vi "CLD 13 Flow Rates Exercise.vi"() -> ()   [LabVIEW 2025]
doc: "CLD 13 exercise"
uses:
  CLD 13 State Machine Enum.ctl
  CLD 13 Data Cluster.ctl
  CLD 13 timer Enum.ctl
panel:
  out "Elapsed Time":dbl
  out "Flow Rate Meter":i8(knob) scale=-20.0..20.0 scale format="%_2f"
  out "Flow Rate":dbl
  out "Error Out":errorcluster
  in  "Error In":errorcluster
  in  "Stop Application":bool
  in  "Stop Flow":bool
  in  "Flow Rate Change":i8(slide) min=-2 max=2 step=1 scale=-2.0..2.0
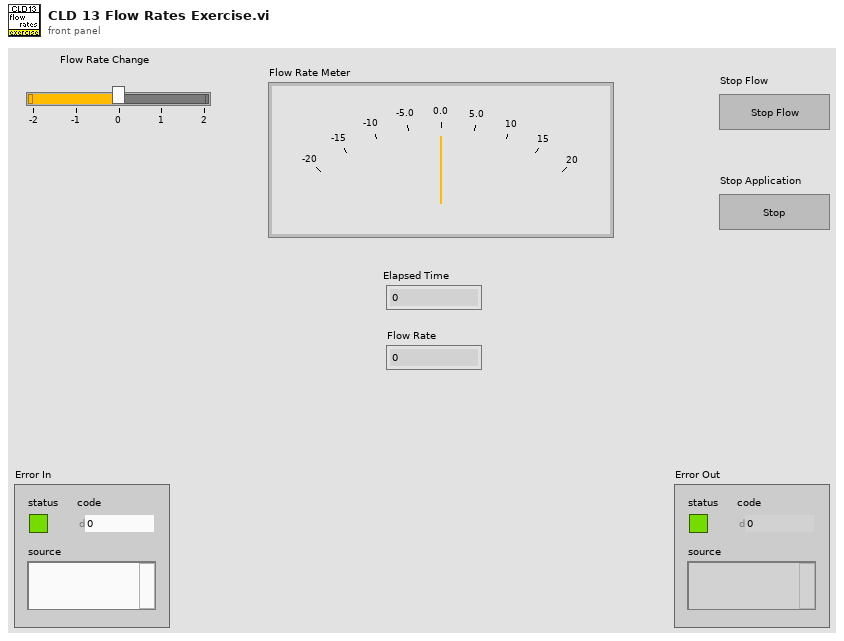
[diagram p1: front panel]
types:
  T1 = typedef "CLD 13 Data Cluster.ctl" = cluster{"Flow Rate Change":i8, "Flow Rate":i8}
  T2 = typedef "CLD 13 State Machine Enum.ctl" = enum16{"Initialize", "Idle", "Stop Flow", "Process"}
  T3 = cluster{"Cluster":T1, "Flow Rate Target":i8, "Operation Mode":enum16{"Normal", "Stop Flow"}}
  T4 = typedef "CLD 13 timer Enum.ctl" = enum16{"Start", "Read"}
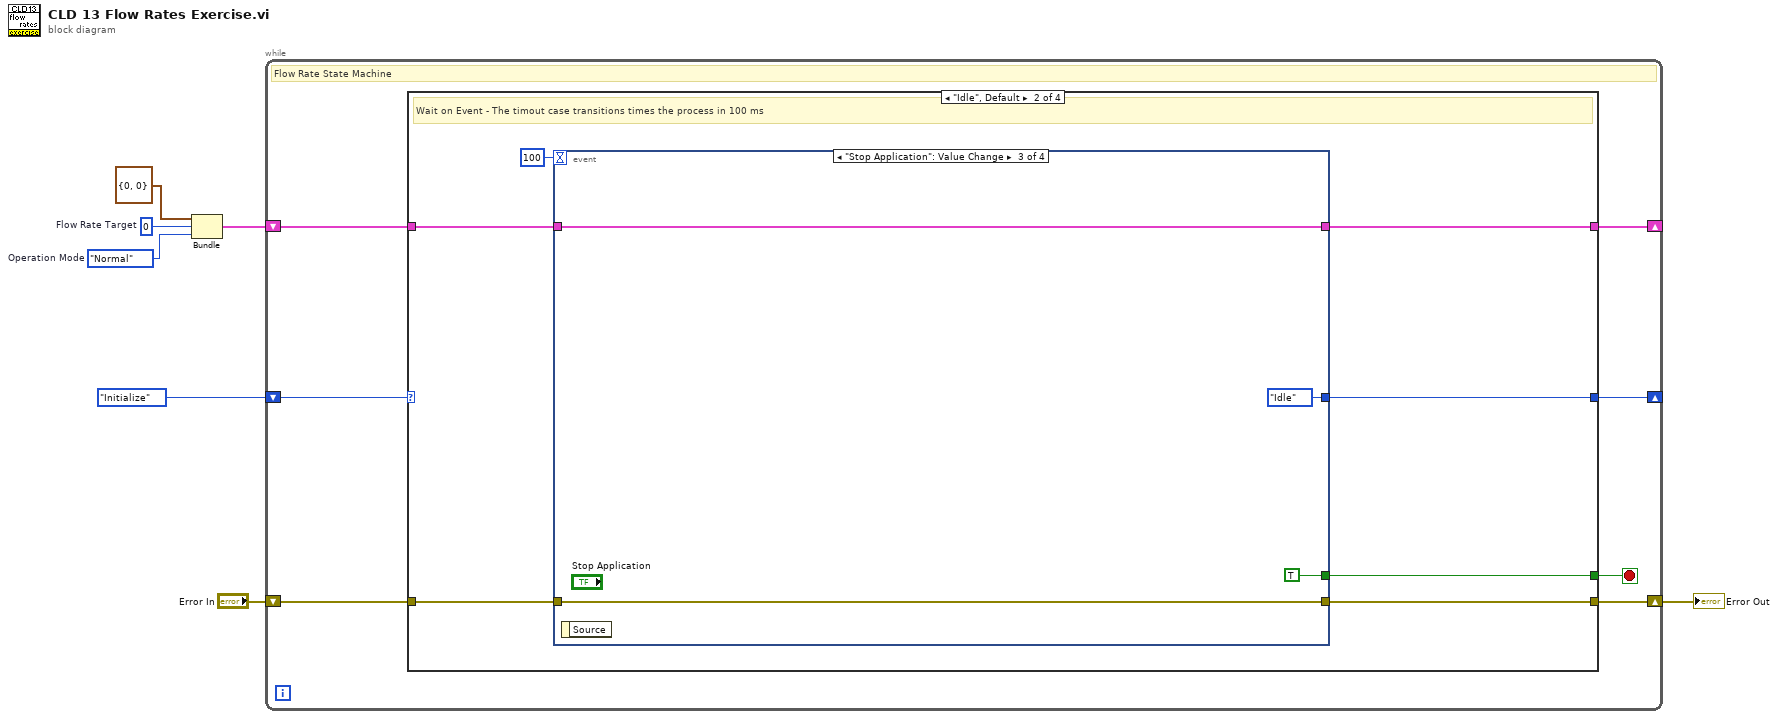
[diagram p0: block diagram]
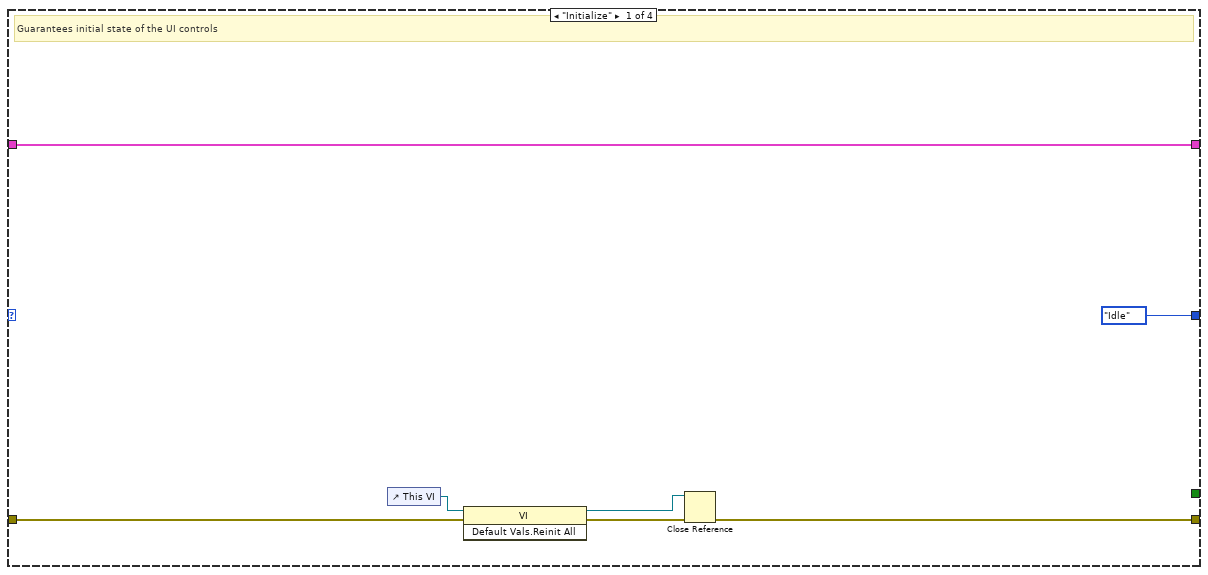
[diagram p2: hidden frame]
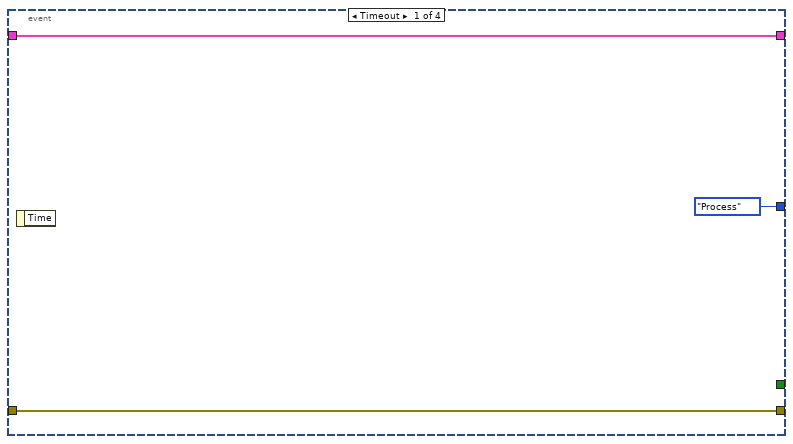
[diagram p3: hidden frame]
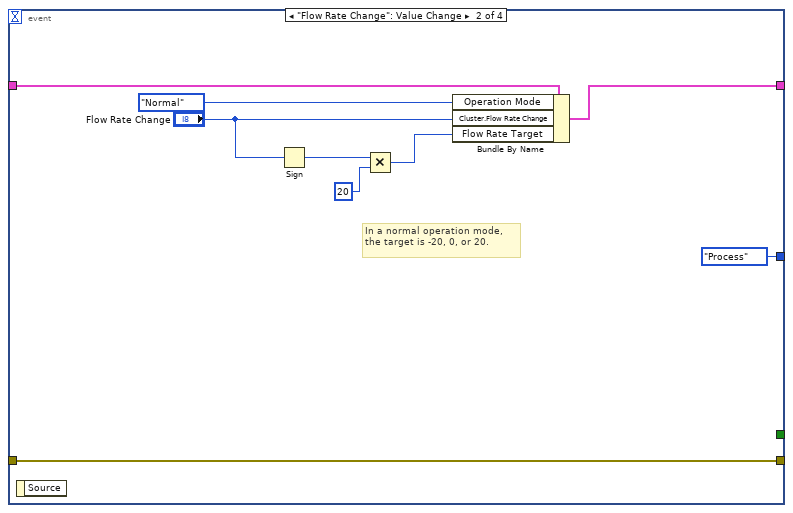
[diagram p4: hidden frame]
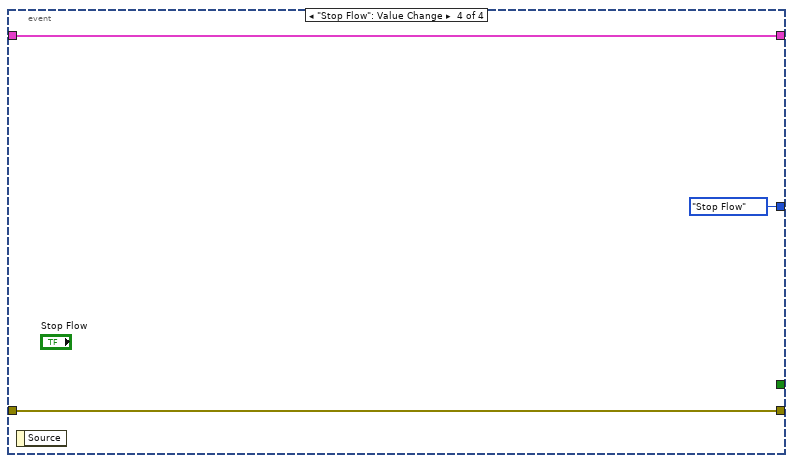
[diagram p5: hidden frame]
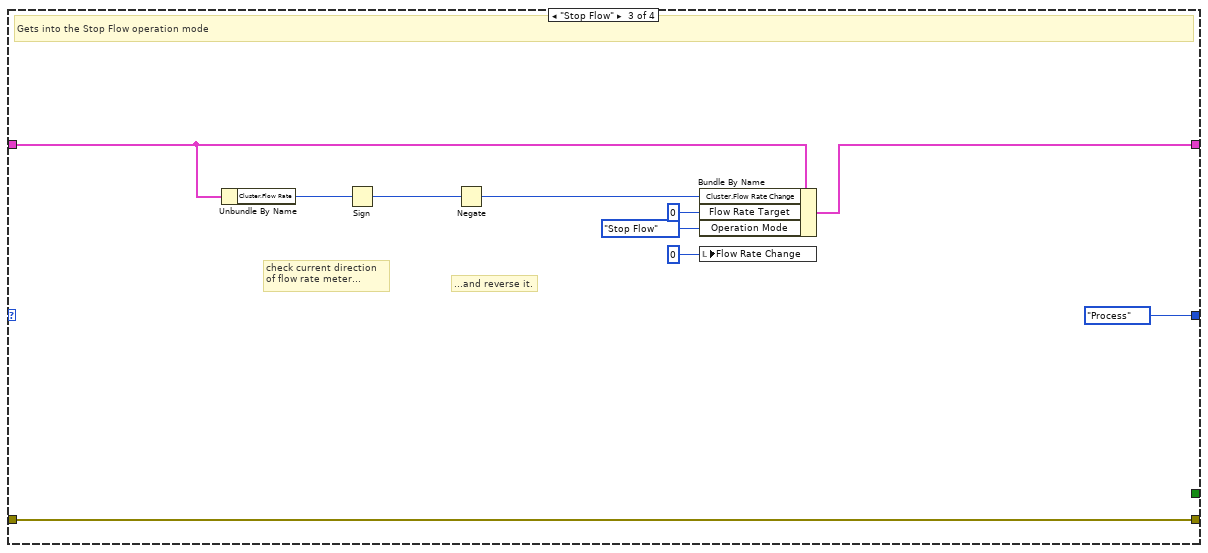
[diagram p6: hidden frame]
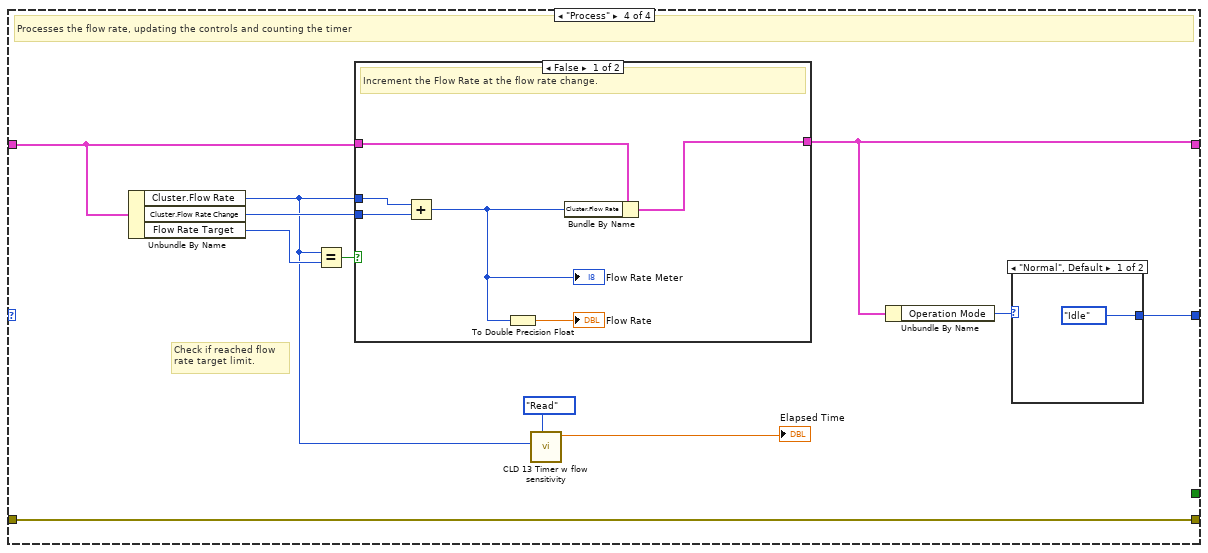
[diagram p7: hidden frame]
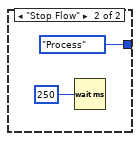
[diagram p8: hidden frame]
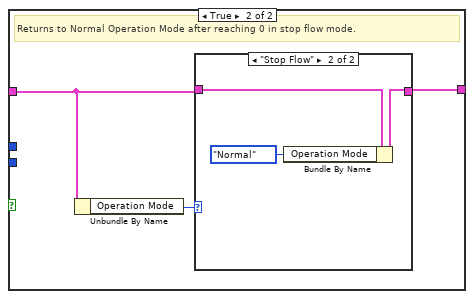
[diagram p9: hidden frame]
diagram:
  w1 = enum16{"Normal", "Stop Flow"}."Normal"  # Operation Mode
  w3 = i8 0  # Flow Rate Target
  n1 = Bundle("Cluster"=T1 {"Flow Rate Change"=0, "Flow Rate"=0}, "Flow Rate Target"=w3, "Operation Mode"=w1) -> (w2:T3)  [unwired: 1 in]
  n2 = while {
    shift-right: [w13] -> w6
    shift-left: "Error In" -> [w14]
    shift-right: [w10] -> _
    shift-left: w2 -> [w11]
    shift-right: [w9] -> _
    shift-left: CLD_13_State_Machine_Enum."Initialize" ("CLD 13") -> [w12]
    stop <- w8 stop-if-true
    # "Flow Rate State Machine"
    n3 = case shown="\"Idle\", Default" w12 {
      tunnel: w14 -> [w21 w28 w57 w68]
      tunnel: [w18 w25 w57 w68] -> w13
      tunnel: w11 -> [w20 w23 w52 w61]
      tunnel: [w20 w26 w51 w62] -> w10
      tunnel: [CLD_13_State_Machine_Enum."Idle" ("CLD 13") w27 CLD_13_State_Machine_Enum."Process" ("CLD 13") w59] -> w9
      tunnel: [_ w24 _ _] -> w8
      frame "Initialize" {
        # "Guarantees initial state of the UI controls"
        n4 = control-ref of="This VI"() -> (w16:refnum<vi>)
        n5 = invoke class="VI" method="Default Vals.Reinit All"(reference=w16, error in=w21) -> (reference out=w17:refnum<vi>, error out=w19:errorcluster)  [unwired: 1 in, 1 out]
        n6 = Close Reference(reference=w17, error in (no error)=w19) -> (error out=w18:errorcluster)
      }
      frame "Idle", Default {
        # "Wait on Event - The timout case transitions times the process in 100 ms"
        n7 = event shown="[2] \"Stop Application\": Value Change" {
          selector: _ -> [_ _ _ _]
          dyn-events: _ -> [_ _ _ _]
          timeout: 100 -> [_ _ _ _]
          tunnel: w28 -> [w31 w38 w44 w47]
          tunnel: w23 -> [w29 w40 w43 w45]
          tunnel: [CLD_13_State_Machine_Enum."Process" ("CLD 13") CLD_13_State_Machine_Enum."Process" ("CLD 13") CLD_13_State_Machine_Enum."Idle" ("CLD 13") CLD_13_State_Machine_Enum."Stop Flow" ("CLD 13")] -> w27
          tunnel: [w29 w39 w43 w45] -> w26
          tunnel: [w31 w38 w44 w47] -> w25
          tunnel: [_ _ TRUE _] -> w24
          event Timeout {
            n8 = event-data() -> ()  [unwired: 1 in, 1 out]
          }
          event "Flow Rate Change": Value Change {
            # "In a normal operation mode, \nthe target is -20, 0, or 20."
            n9 = event-data() -> ()  [unwired: 1 in, 1 out]
            n10 = Sign(1:"Flow Rate Change") -> (0:w34:i8)
            n11 = Multiply(x=w34, y=i8 20) -> (x*y=w32:i8)
            n12 = Bundle By Name(cluster=w40, "Operation Mode"=enum16{"Normal", "Stop Flow"}."Normal", "Cluster.Flow Rate Change"="Flow Rate Change", "Flow Rate Target"=w32) -> (w39:T3)
          }
          event "Stop Application": Value Change {
            n13 = event-data() -> ()  [unwired: 1 in, 1 out]
          }
          event "Stop Flow": Value Change {
            n14 = event-data() -> ()  [unwired: 1 in, 1 out]
          }
        }
      }
      frame "Stop Flow" {
        # "...and reverse it."
        # "check current direction\nof flow rate meter..."
        # "Gets into the Stop Flow operation mode"
        n15 = Unbundle By Name(w52) -> ("Cluster.Flow Rate"=w56:i8)
        n16 = Sign(1:w56) -> (0:w55:i8)
        n17 = Negate(x=w55) -> (-x=w54:i8)
        n18 = Bundle By Name(cluster=w52, "Cluster.Flow Rate Change"=w54, "Flow Rate Target"=i8 0, "Operation Mode"=enum16{"Normal", "Stop Flow"}."Stop Flow") -> (w51:T3)
        n19 = local write "Flow Rate Change"(i8 0 ("Flow Rate Change")) -> ()
      }
      frame "Process" {
        # "Check if reached flow\nrate target limit."
        # "Processes the flow rate, updating the controls and counting the timer"
        n20 = Unbundle By Name(w61) -> ("Cluster.Flow Rate"=w58:i8, "Cluster.Flow Rate Change"=w67:i8, "Flow Rate Target"=w66:i8)
        n21 = Equal?(x=w58, y=w66) -> (x = y?=w65:bool)
        n22 = case shown="False" w65 {
          tunnel: w61 -> [w77 w79]
          tunnel: [w76 w78] -> w62
          tunnel: w67 -> [w75 _]
          tunnel: w58 -> [w74 _]
          frame False {
            # "Increment the Flow Rate at the flow rate change."
            n23 = Add(x=w74, y=w75) -> (x+y=w72:i8)
            "Flow Rate Meter" <- w72
            n24 = To Double Precision Float(number=w72) -> (double precision float=→"Flow Rate":dbl)
            n25 = Bundle By Name(cluster=w77, "Cluster.Flow Rate"=w72) -> (w76:T3)
          }
          frame True {
            # "Returns to Normal Operation Mode after reaching 0 in stop flow mode."
            n26 = Unbundle By Name(w79) -> ("Operation Mode"=w80:enum16{"Normal", "Stop Flow"})
            n27 = case shown="\"Stop Flow\"" w80 {
              tunnel: w79 -> [w81 w84]
              tunnel: [w81 w83] -> w78
              frame "Normal", Default {
              }
              frame "Stop Flow" {
                n28 = Bundle By Name(cluster=w84, "Operation Mode"=enum16{"Normal", "Stop Flow"}."Normal") -> (w83:T3)
              }
            }
          }
        }
        n29 = call "CLD 13 Timer w flow sensitivity.vi"("Flow Rate"=w58, "Timer Enum"=CLD_13_timer_Enum."Read") -> ("Time elapsed"=→"Elapsed Time":dbl)  [unwired: 8 in, 1 out]
        n30 = Unbundle By Name(w62) -> ("Operation Mode"=w60:enum16{"Normal", "Stop Flow"})
        n31 = case shown="\"Normal\", Default" w60 {
          tunnel: [CLD_13_State_Machine_Enum."Idle" ("CLD 13") CLD_13_State_Machine_Enum."Process" ("CLD 13")] -> w59
          frame "Normal", Default {
          }
          frame "Stop Flow" {
            n32 = Wait (ms)(milliseconds to wait=u32 250) -> ()  [unwired: 1 out]
          }
        }
      }
    }
  }
  "Error Out" <- w6
